vi "change alarm operation.vi"(8 "error in":errorcluster, 9 "boolean op":T1, 10 "alarm name":string, 11 "alarms module configuration in":refnum<class "alarms module configuration.lvclass">) -> (0 "error out":errorcluster, 3 "alarms module configuration out":refnum<class "alarms module configuration.lvclass">)   [LabVIEW 2013, in "alarms module configuration.lvclass"]
uses:
  alarms module configuration.lvclass
  boolean operation.ctl
  alarms module configuration.lvclass/alarms module configuration.ctl
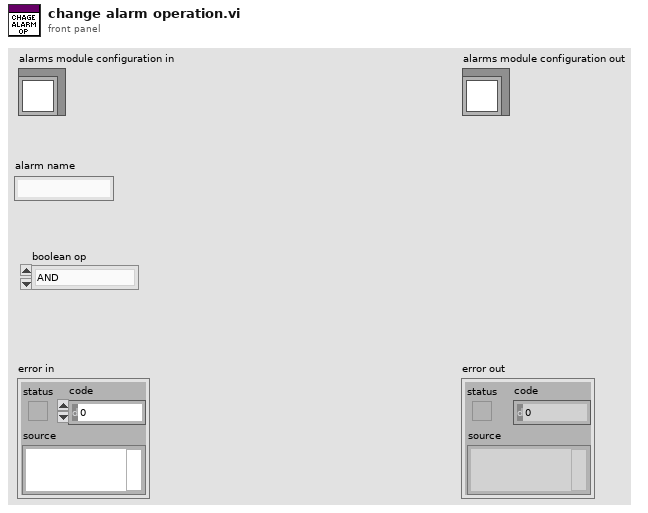
[diagram p1: front panel]
types:
  T1 = typedef "alarms module configuration.lvclass/boolean operation.ctl" = enum16{"AND", "OR"}
  T2 = typedef "alarms module configuration.lvclass/alarm configuration.ctl" = cluster{"alarm name":string, "comparisons":T3[], "unlatch":refnum<class "TBM channel.lvclass">, "output":refnum<class "TBM channel.lvclass">, "boolean op":T1}
  T3 = typedef "alarms module configuration.lvclass/alarm comparison.ctl" = cluster{"input channel":refnum<class "TBM channel.lvclass">, "limit":dbl, "comparison":T4}
  T4 = typedef "alarms module configuration.lvclass/compare type.ctl" = enum16{">", "<", ">=", "<=", "="}
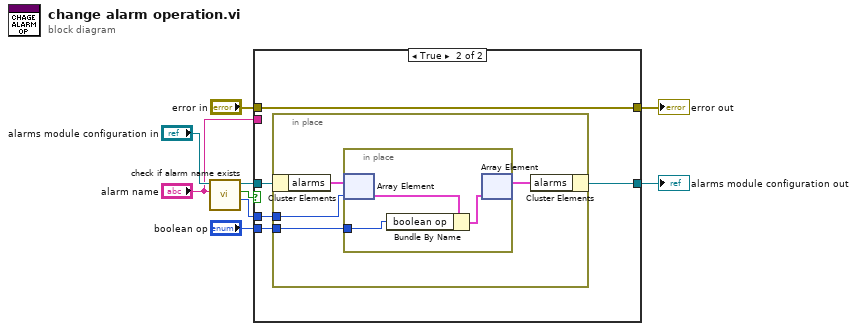
[diagram p0: block diagram]
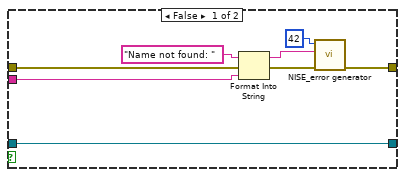
[diagram p2: hidden frame]
diagram:
  n1 = call "check if alarm name exists.vi"("name to locate"="alarm name", "alarms module configuration in"="alarms module configuration in") -> ("index"=w3:i32, "found?"=w6:bool, "alarms module configuration out"=w4:refnum<class "alarms module configuration.lvclass">)  [unwired: 6 in, 1 out]
  n2 = case shown="True" w6 {
    tunnel: [w16 w20] -> w8
    tunnel: "error in" -> [w17 w20]
    tunnel: [w11 w21] -> w5
    tunnel: w4 -> [w11 w22]
    tunnel: w3 -> [_ w19]
    tunnel: "alarm name" -> [w10 _]
    tunnel: "boolean op" -> [_ w18]
    frame False {
      n3 = Format Into String(initial string="Name not found: " ("append error message"), error in=w17, w10) -> (resulting string=w12:string, error out=w14:errorcluster)  [unwired: 1 in]
      n4 = call <vilib>:"NISE_error generator.vi"("error in"=w14, "append error message"=w12, "error code (0)"=42) -> ("error out"=w16:errorcluster)  [unwired: 6 in]
    }
    frame True {
      n5 = in-place {
        in-place-border: w19 -> [w24]
        in-place-border: w18 -> [w23]
        n6 = in-place-cluster #1(w22) -> ("alarms"=w26:T2[])
        n7 = in-place {
          in-place-border: w23 -> [w27]
          n8 = in-place-array #2(w26, w24) -> (w29:T2)
          n9 = Bundle By Name(cluster=w29, "boolean op"=w27) -> (w28:T2)
          n10 = in-place-array #2(w28) -> (w25:T2[])  [unwired: 1 out]
        }
        n11 = in-place-cluster #1("alarms"=w25) -> (w21:refnum<class "alarms module configuration.lvclass">)
      }
    }
  }
  "error out" <- w8
  "alarms module configuration out" <- w5
